vi "Teleop.vi"(10 "Match Info":T2={"Autonomous Elapsed Seconds"=0.0, "TeleOp Elapsed Seconds"=0.0, "Disabled Elapsed Seconds"=0.0, "Visited Autonomous"=FALSE, "Visited TeleOp"=FALSE, "Visited Disabled"=FALSE, "Autonomous Settings"={"Autonomous Style"=enum."Independent", "VI Refnum"=refnum}}, 11 "Call Context":T3) -> ()   [LabVIEW 2017]
doc: "This VI is called for each enabled TeleOp packet received from the DS. It is typically used to read from joysticks and other inputs and update I/O or setpoints for timed control loops. It should complete and return within 20 milliseconds or risk missing DS packets."
uses:
  <vilib>/Rock Robotics/WPI/DriverStation/WPI_DriverStationDerivedRobotMode.ctl
  <vilib>/Rock Robotics/WPI/DriverStation/WPI_DriverStationMatch Info.ctl
  <vilib>/Rock Robotics/WPI/Utilities/WPI_GetSetVariantRefNum.vi
  <vilib>/Rock Robotics/Network Tables/NT Write Boolean Array.vi
  <vilib>/Rock Robotics/Network Tables/NT Write Numeric Array.vi
  Framework/Robot Global Data.vi
panel:
  in  "n^x(Unbounded)":dbl=2.5 format="%#_13g"
  in  "Select Function":T1(ring)=enum."Square"
  in  "Dead Zone(0 to 1)":dbl=0.01
  in  "Min Output(0 to 1)":dbl=0.1
  in  "Turn Rate":dbl=1.0
  in  "Speed Rate":dbl=1.0
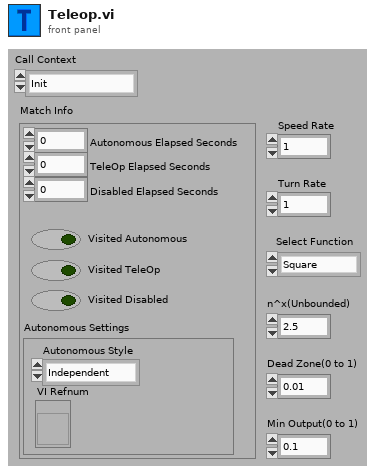
[diagram p1: front panel]
types:
  T1 = enum16{"Linear", "Square  Root", "Square", "n^x"}
  T2 = typedef "WPI_DriverStationMatch Info.ctl" = cluster{"Autonomous Elapsed Seconds":dbl, "TeleOp Elapsed Seconds":dbl, "Disabled Elapsed Seconds":dbl, "Visited Autonomous":bool, "Visited TeleOp":bool, "Visited Disabled":bool, "Autonomous Settings":cluster{"Autonomous Style":enum16{"Iterative", "Independent"}, "VI Refnum":refnum<vi>}}
  T3 = typedef "WPI_DriverStationDerivedRobotMode.ctl" = enum16{"Init", "Execute", "Stop"}
  T4 = typedef "WPI_JoystickDevRef.ctl" = cluster{"Device":T5}
  T5 = typedef "WPI_JoystickDeviceEnum.ctl" = enum16{"USB 0", "USB 1", "USB 2", "USB 3", "USB 4", "USB 5"}
  T6 = cluster{"X":dbl, "Y":dbl, "Angle":dbl, "Magnitude":dbl}
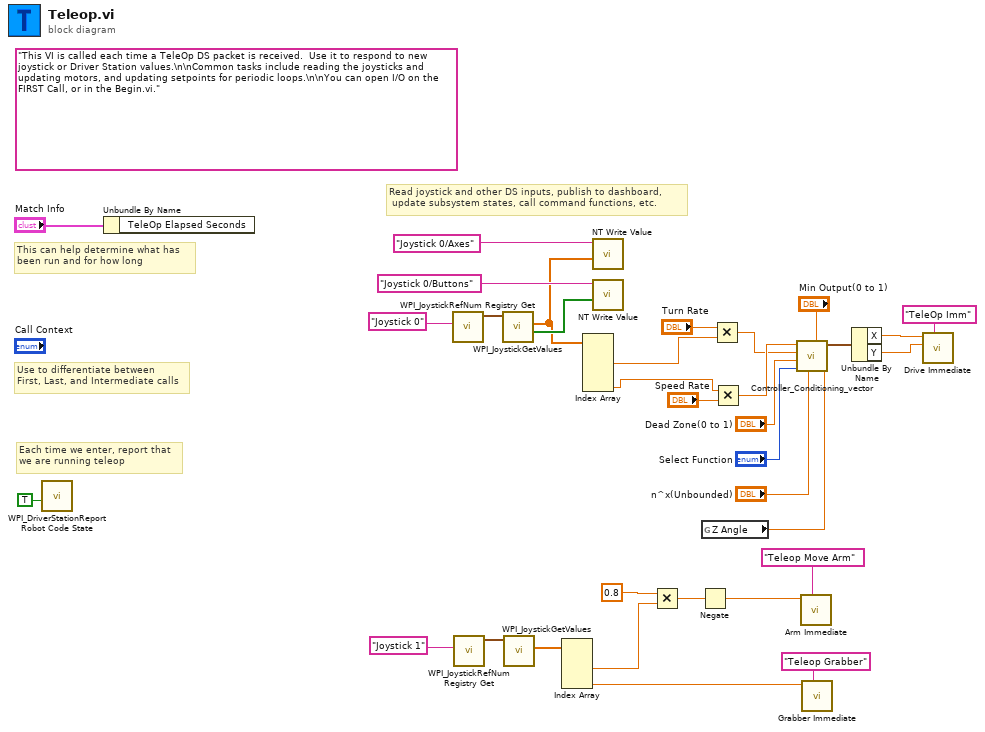
[diagram p0: block diagram]
diagram:
  (unwired) "This VI is called each time a TeleOp DS packet is received.  Use it to respond to new joystick or Driver Station values.\n\nCommon tasks include reading the joysticks and updating motors, and updating setpoints for periodic loops.\n\nYou can open I/O on the FIRST Call, or in the Begin.vi."
  # "Read joystick and other DS inputs, publish to dashboard,\n update subsystem states, call command functions, etc."
  # "Each time we enter, report that\nwe are running teleop"
  # "Use to differentiate between\nFirst, Last, and Intermediate calls"
  # "This can help determine what has\nbeen run and for how long"
  n1 = call <vilib>:"WPI_DriverStationReport Robot Code State.vi"("TeleOp"=TRUE ("Autonomous")) -> ()  [unwired: 10 in, 1 out]
  n2 = Unbundle By Name("Match Info") -> ()  [unwired: 1 out]
  n3 = call <vilib>:"WPI_JoystickRefNum Registry Get.vi"("refnum name"="Joystick 0") -> ("JoystickDevRef"=w30:T4)  [unwired: 1 in, 9 out]
  n4 = call <vilib>:"WPI_JoystickRefNum Registry Get.vi"("refnum name"="Joystick 1") -> ("JoystickDevRef"=w25:T4)  [unwired: 1 in, 9 out]
  n5 = call <vilib>:"WPI_JoystickGetValues.vi"("JoystickDevRef"=w30) -> ("Buttons"=w27:bool[], "Axes"=w17:dbl[])  [unwired: 6 in, 3 out]
  n6 = call <vilib>:"WPI_JoystickGetValues.vi"("JoystickDevRef"=w25) -> ("Axes"=w13:dbl[])  [unwired: 6 in, 4 out]
  n7 = Index Array(array=w13) -> (element #2=w16:dbl, element #4=w12:dbl)  [unwired: 4 in, 2 out]
  n8 = Index Array(array=w17) -> (element #2=w18:dbl, element #5=w19:dbl)  [unwired: 5 in, 3 out]
  n9 = call-poly <vilib>:"NT Write Value.vi"("Numeric Array"=w17, "Name"="Joystick 0/Axes") -> ()  [unwired: 9 in, 1 out]
  n10 = call-poly <vilib>:"NT Write Value.vi"("Boolean Array"=w27, "Name"="Joystick 0/Buttons") -> ()  [unwired: 9 in, 1 out]
  n11 = Multiply(x=0.8, y=w16) -> (x*y=w14:dbl)
  n12 = Negate(x=w14) -> (-x=w11:dbl)
  n13 = global read "Robot Global Data.vi" "Z Angle"() -> (w5:dbl)
  n14 = Multiply(x="Turn Rate", y=w18) -> (x*y=w9:dbl)
  n15 = Multiply(x=w19, y="Speed Rate") -> (x*y=w10:dbl)
  n16 = call "Controller_Conditioning_vector.vi"("Angular Offset\n(-180 to 180 or 0 to 360)"=w5, "Min Output(0 to 1)"="Min Output(0 to 1)", "n^x(Unbounded)"="n^x(Unbounded)", "Select Function"="Select Function", "Dead Zone(0 to 1)"="Dead Zone(0 to 1)", "Y(-1 to 1)"=w9, "X(-1 to 1)"=w10) -> ("output cluster"=w8:T6)  [unwired: 4 in]
  n17 = call "Arm Immediate.vi"("Description"="Teleop Move Arm", "Setpoint"=w11) -> ()  [unwired: 9 in, 1 out]
  n18 = call "Grabber Immediate.vi"("Description"="Teleop Grabber", "Setpoint"=w12) -> ()  [unwired: 9 in, 1 out]
  n19 = Unbundle By Name(w8) -> ("X"=w7:dbl, "Y"=w6:dbl)
  n20 = call "Drive Immediate.vi"("Description"="TeleOp Imm", "Right Setpoint"=w6, "Left Setpoint"=w7) -> ()  [unwired: 8 in, 1 out]
